vi "TrendsD06.vi"() -> ()   [LabVIEW 2019, in "D06.lvlib"]
uses:
  D06.lvlib
  <vilib>/measure/mamon.llb/Trigger Detection for 1 Channel.vi
  <vilib>/measure/NI_MAPro.lvlib
panel:
  out "No Change":bool
  out "Sudden Change":bool
  out "Decrease":bool
  out "Increase":bool
  out "Previous  ES":dbl
  out "Present  Speed":dbl
  out "Present Error":dbl format="%#.2g"
  out "Previous Error":dbl
  out "Previous  Speed":dbl
  out "Previous PW":dbl caption="Control Information"
  out "Pulse Trends":waveform(i16)[](graph) caption="Waveform Chart - Dark"
  in  "Close":bool
  out "disc name":string="Disc 06 Trends"
  out "dsgs":string="DSGS"
  out "Speed Trend":waveform(dbl)(graph) caption="Waveform Chart - Dark"
  out "Average Trend":waveform(dbl)[](graph) caption="Waveform Chart - Dark"
  out "Live Trend":waveform(dbl)[](graph) caption="Waveform Chart - Dark"
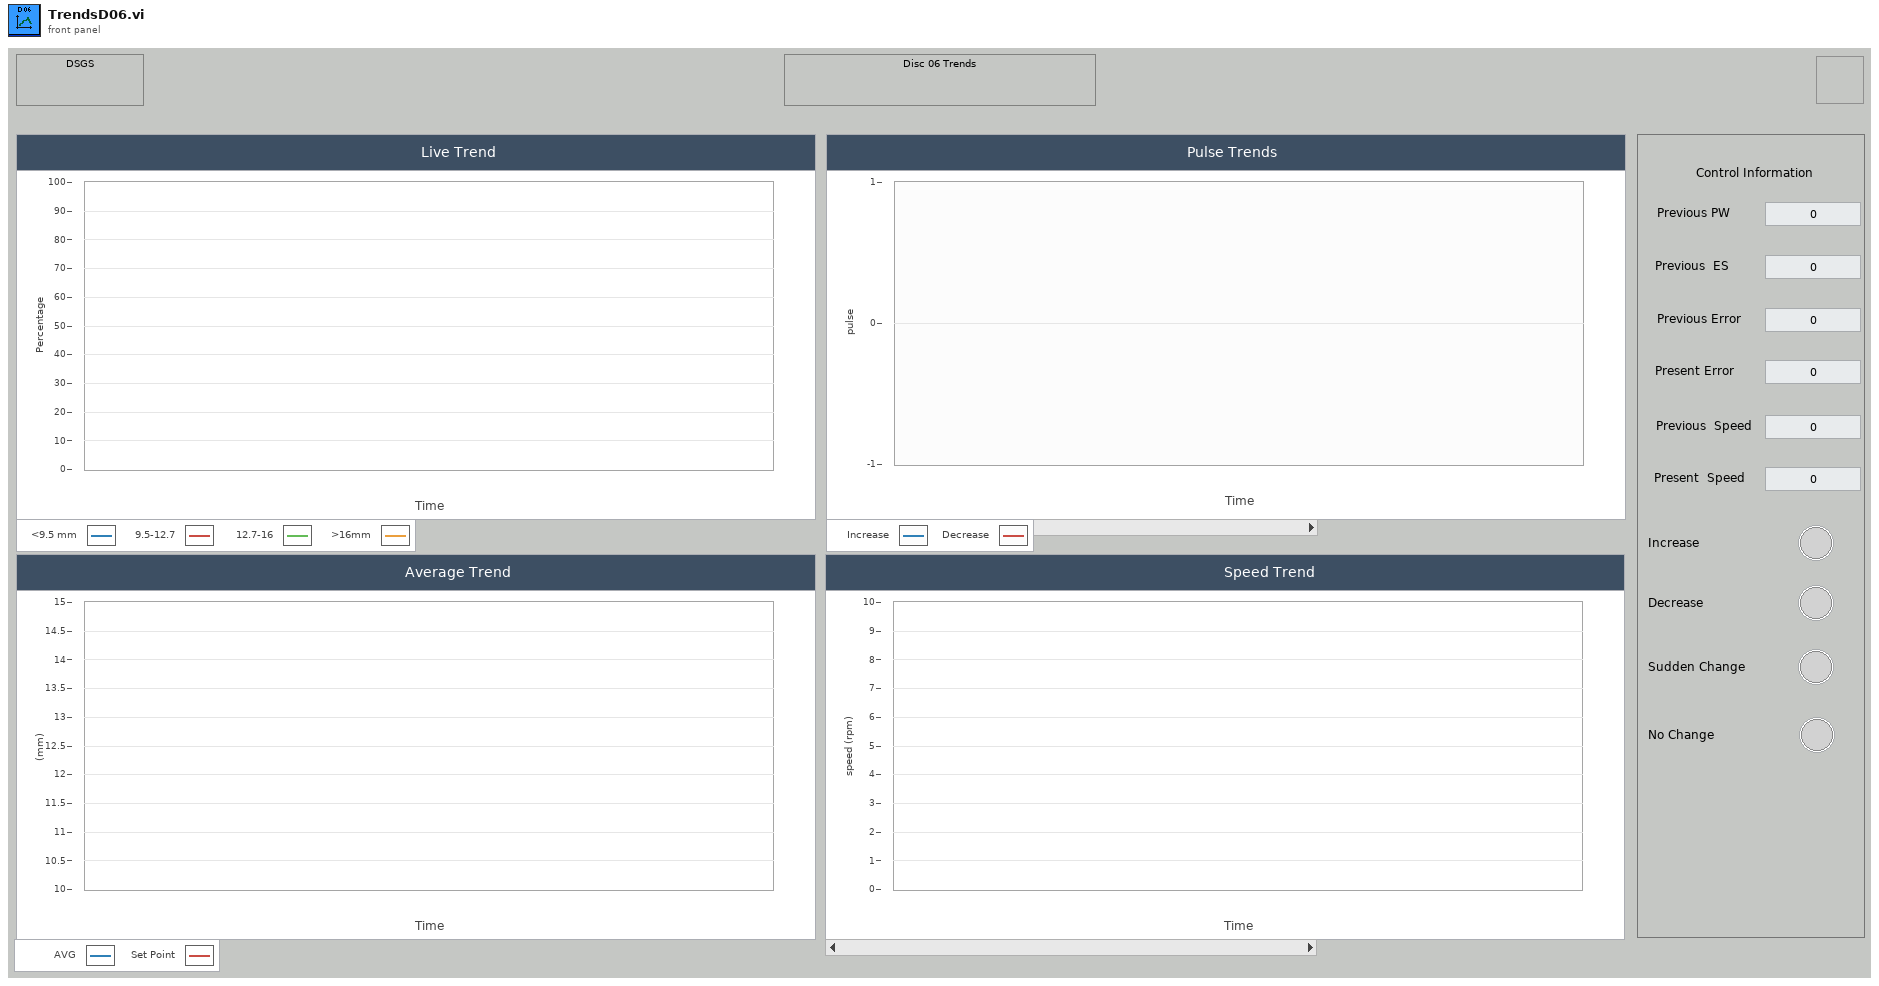
[diagram p1: front panel]
types:
  T1 = cluster{"decrease D06":bool, "increase D06":bool, "no change D06":bool, "sudden change D06":bool, "last error 06":dbl, "previouse speed D06":dbl, "pulse width D06":dbl, "slope D06":dbl}
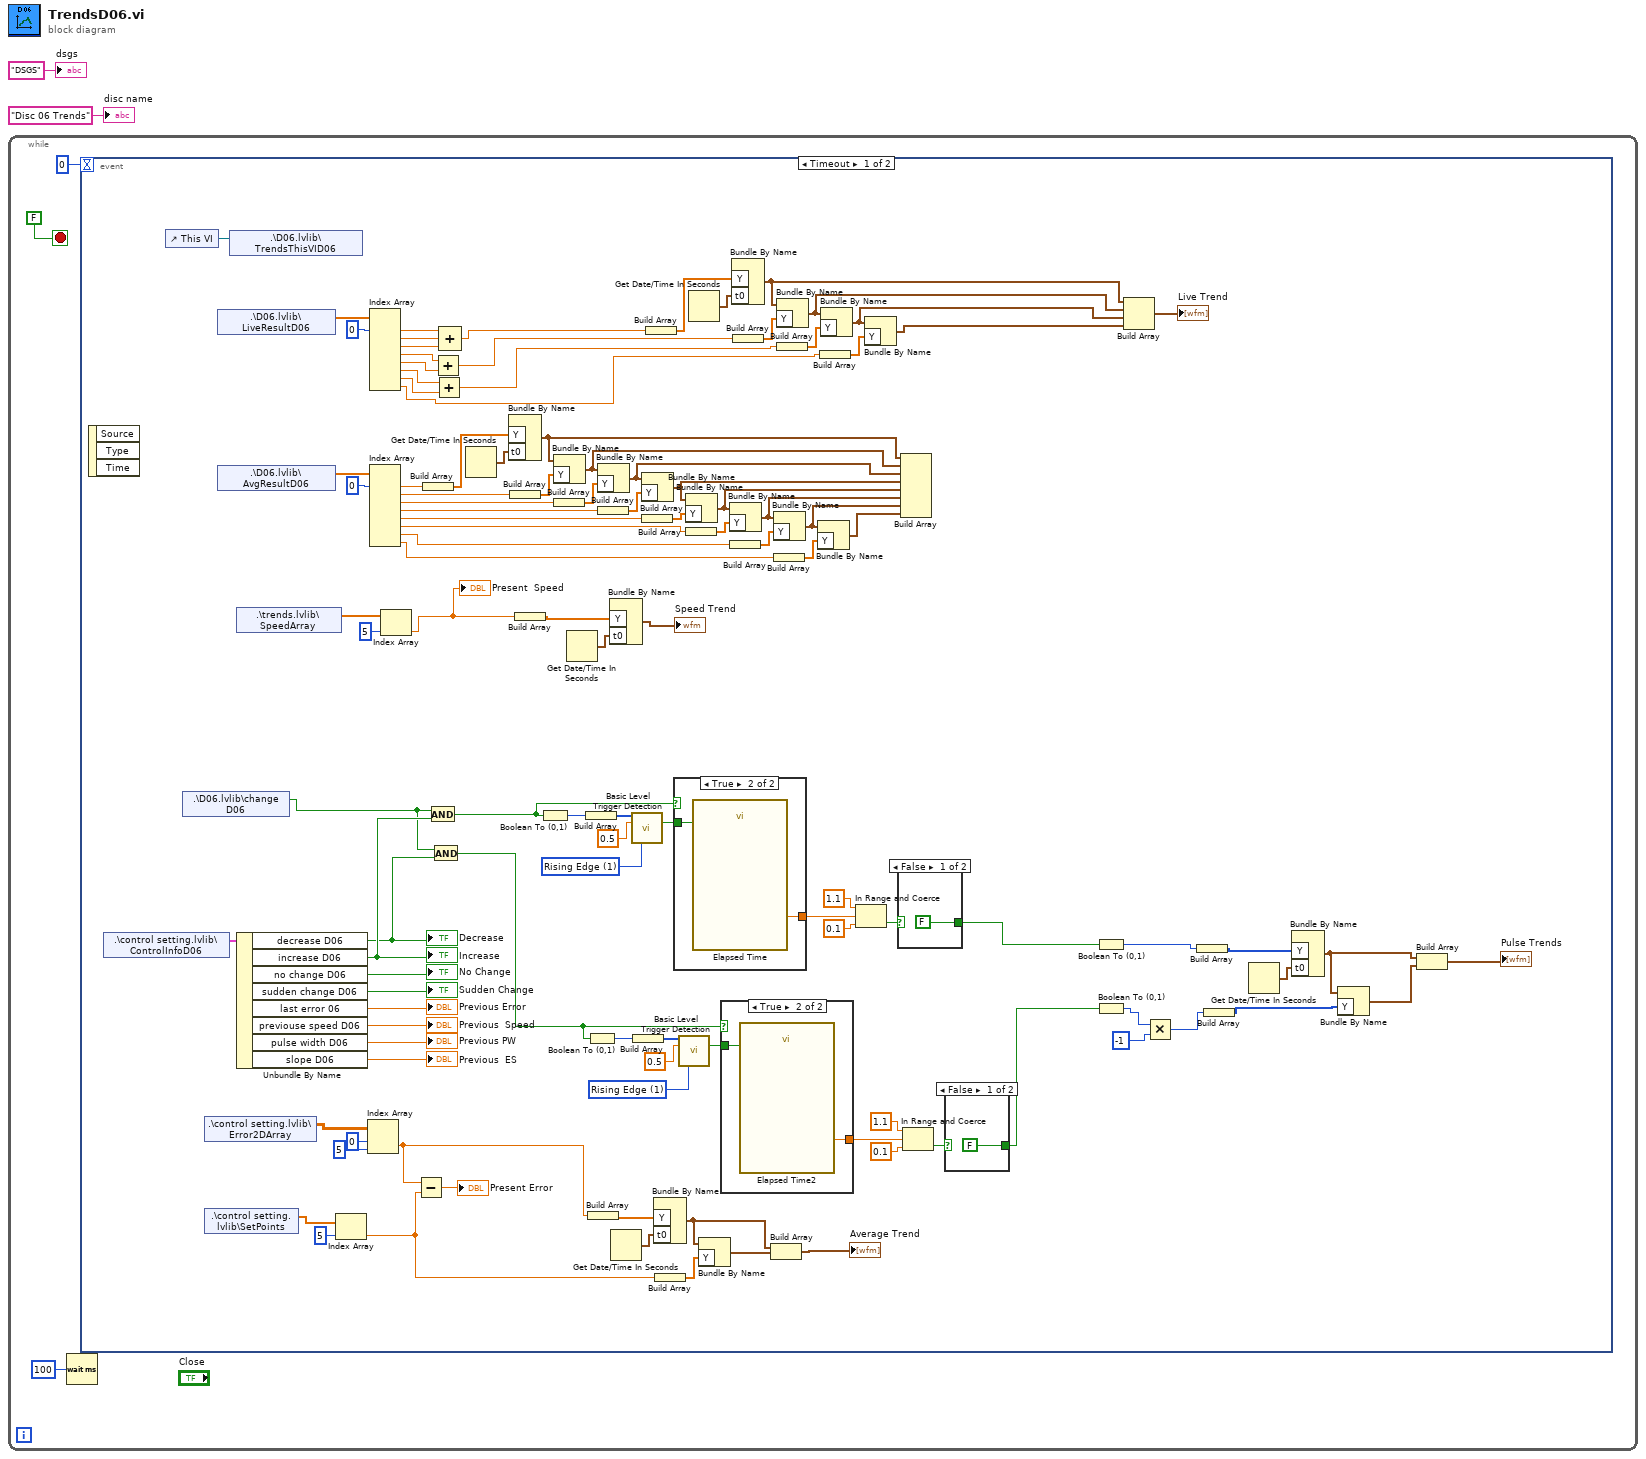
[diagram p0: block diagram]
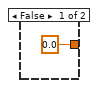
[diagram p2: hidden frame]
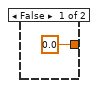
[diagram p4: hidden frame]
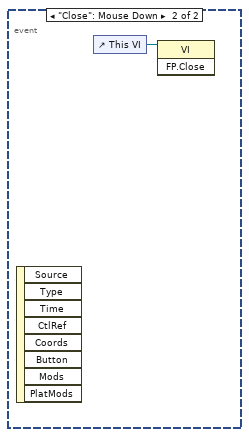
[diagram p6: hidden frame]
diagram:
  n1 = while {
    stop <- FALSE stop-if-true
    n2 = Wait (ms)(milliseconds to wait=u32 100) -> ()  [unwired: 1 out]
    n3 = event shown="[0] Timeout" {
      selector: _ -> [_ _]
      dyn-events: _ -> [_ _]
      timeout: 0 -> [_ _]
      event Timeout {
        w30 = u16 1 items=["Falling Edge", "Rising Edge"] ("trigger slope")
        w42 = u16 1 items=["Falling Edge", "Rising Edge"] ("trigger slope")
        n4 = event-data() -> ()  [unwired: 1 in, 3 out]
        n5 = shared-variable ".\\control setting.lvlib\\ControlInfoD06"() -> (w63:T1)  [unwired: 1 in, 1 out]
        n6 = control-ref of="This VI"() -> (w79:refnum<vi>)
        n7 = shared-variable ".\\D06.lvlib\\change D06"() -> (w28:bool)  [unwired: 1 in, 1 out]
        n8 = shared-variable ".\\control setting.lvlib\\Error2DArray"() -> (w56:dbl[][])  [unwired: 1 in, 1 out]
        n9 = shared-variable ".\\control setting.lvlib\\SetPoints"() -> (w53:dbl[])  [unwired: 1 in, 1 out]
        n10 = shared-variable ".\\D06.lvlib\\LiveResultD06"() -> (w118:dbl[])  [unwired: 1 in, 1 out]
        n11 = shared-variable ".\\D06.lvlib\\AvgResultD06"() -> (w85:dbl[])  [unwired: 1 in, 1 out]
        n12 = shared-variable ".\\D06.lvlib\\TrendsThisVID06"(w79) -> ()  [unwired: 1 in, 1 out]
        n13 = shared-variable ".\\trends.lvlib\\SpeedArray"() -> (w68:dbl[])  [unwired: 1 in, 1 out]
        n14 = Unbundle By Name(w63) -> ("decrease D06"=w27:bool, "increase D06"=w40:bool, "no change D06"=→"No Change":bool, "sudden change D06"=→"Sudden Change":bool, "last error 06"=→"Previous Error":dbl, "previouse speed D06"=→"Previous  Speed":dbl, "pulse width D06"=→"Previous PW":dbl, "slope D06"=→"Previous  ES":dbl)
        "Increase" <- w40
        "Decrease" <- w27
        n15 = Index Array(array=w53, index=5) -> (element=w9:dbl)
        n16 = Index Array(array=w56, index (row)=0, index (col)=5 ("disabled index (col)")) -> (element=w10:dbl)
        n17 = Index Array(array=w118, index #1=0 ("index")) -> (element #1=w24:dbl, element #2=w23:dbl, element #3=w22:dbl, element #4=w21:dbl, element #5=w20:dbl, element #6=w19:dbl, element #7=w18:dbl, element #8=w14:dbl)  [unwired: 7 in]
        n18 = Index Array(array=w85, index #1=0 ("index")) -> (element #1=w95:dbl, element #2=w96:dbl, element #3=w98:dbl, element #4=w100:dbl, element #5=w101:dbl, element #6=w103:dbl, element #7=w105:dbl, element #8=w82:dbl)  [unwired: 7 in]
        n19 = Index Array(array=w68, index=5) -> (element=w50:dbl)
        "Present  Speed" <- w50
        n20 = Subtract(x=w10, y=w9) -> (x-y=→"Present Error":dbl)
        n21 = Build Array(w95) -> (w106:dbl[])
        n22 = And(x=w28, y=w40) -> (x .and. y?=w39:bool)
        n23 = And(x=w28, y=w27) -> (x .and. y?=w26:bool)
        n24 = Add(x=w21, y=w20) -> (x+y=w16:dbl)
        n25 = Add(x=w19, y=w18) -> (x+y=w15:dbl)
        n26 = Compound Arithmetic op=ADD(w24, w23, w22) -> (w17:dbl)
        n27 = Get Date/Time In Seconds() -> (seconds since 1Jan1904=w88:timestamp)
        n28 = Bundle By Name("Y"=w106, "t0"=w88) -> (w94:waveform(dbl))  [unwired: 1 in]
        n29 = Build Array(w96) -> (w97:dbl[])
        n30 = Build Array(w50) -> (w66:dbl[])
        n31 = Boolean To (0,1)(Boolean=w39) -> (0, 1=w45:i16)
        n32 = Bundle By Name(cluster=w94, "Y"=w97) -> (w93:waveform(dbl))
        n33 = Build Array(w98) -> (w99:dbl[])
        n34 = Get Date/Time In Seconds() -> (seconds since 1Jan1904=w65:timestamp)
        n35 = Build Array(w45) -> (w44:i16[])
        n36 = Boolean To (0,1)(Boolean=w26) -> (0, 1=w33:i16)
        n37 = Build Array(w10) -> (w11:dbl[])
        n38 = Bundle By Name(cluster=w93, "Y"=w99) -> (w92:waveform(dbl))
        n39 = Build Array(w100) -> (w87:dbl[])
        n40 = Bundle By Name("Y"=w66, "t0"=w65) -> (→"Speed Trend":waveform(dbl))  [unwired: 1 in]
        n41 = Get Date/Time In Seconds() -> (seconds since 1Jan1904=w13:timestamp)
        n42 = call-poly <vilib>:"Basic Level Trigger Detection.vi"("signal in"=w44, "level"=0.5, "trigger slope"=w42) -> ("trigger detected?"=w41:bool)  [unwired: 10 in, 2 out]
        n43 = Build Array(w33) -> (w32:i16[])
        n44 = Bundle By Name(cluster=w92, "Y"=w87) -> (w91:waveform(dbl))
        n45 = Build Array(w101) -> (w102:dbl[])
        n46 = Build Array(w17) -> (w108:dbl[])
        n47 = Bundle By Name("Y"=w11, "t0"=w13) -> (w7:waveform(dbl))  [unwired: 1 in]
        n48 = Build Array(w9) -> (w12:dbl[])
        n49 = case shown="True" w39 {
          tunnel: [0.0 ("Elapsed Time (s)") w125] -> w49
          tunnel: w41 -> [_ w126]
          frame False {
          }
          frame True {
            n50 = call "Elapsed Time"("Reset"=w126) -> ("Elapsed Time (s)"=w125:dbl)  [unwired: 11 in, 7 out]
          }
        }
        n51 = call-poly <vilib>:"Basic Level Trigger Detection.vi"("signal in"=w32, "level"=0.5, "trigger slope"=w30) -> ("trigger detected?"=w29:bool)  [unwired: 10 in, 2 out]
        n52 = Bundle By Name(cluster=w91, "Y"=w102) -> (w90:waveform(dbl))
        n53 = Build Array(w103) -> (w104:dbl[])
        n54 = Get Date/Time In Seconds() -> (seconds since 1Jan1904=w115:timestamp)
        n55 = Bundle By Name(cluster=w7, "Y"=w12) -> (w8:waveform(dbl))
        n56 = case shown="True" w26 {
          tunnel: [0.0 ("Elapsed Time (s)") w120] -> w37
          tunnel: w29 -> [_ w121]
          frame False {
          }
          frame True {
            n57 = call "Elapsed Time2"("Reset"=w121) -> ("Elapsed Time (s)"=w120:dbl)  [unwired: 11 in, 7 out]
          }
        }
        n58 = Bundle By Name(cluster=w90, "Y"=w104) -> (w89:waveform(dbl))
        n59 = Build Array(w105) -> (w107:dbl[])
        n60 = Bundle By Name("Y"=w108, "t0"=w115) -> (w111:waveform(dbl))  [unwired: 1 in]
        n61 = Build Array(w16) -> (w110:dbl[])
        n62 = Build Array(w7, w8) -> (→"Average Trend":waveform(dbl)[])
        n63 = Bundle By Name(cluster=w89, "Y"=w107) -> (w83:waveform(dbl))
        n64 = Build Array(w82) -> (w84:dbl[])
        n65 = Bundle By Name(cluster=w111, "Y"=w110) -> (w112:waveform(dbl))
        n66 = Build Array(w15) -> (w109:dbl[])
        n67 = Bundle By Name(cluster=w83, "Y"=w84) -> (w81:waveform(dbl))
        n68 = Build Array(w14) -> (w116:dbl[])
        n69 = Bundle By Name(cluster=w112, "Y"=w109) -> (w113:waveform(dbl))
        n70 = In Range and Coerce(upper limit=1.1, x=w49, lower limit=0.1) -> (In Range?=w46:bool)  [unwired: 1 out]
        n71 = Bundle By Name(cluster=w113, "Y"=w116) -> (w114:waveform(dbl))
        n72 = case shown="False" w46 {
          selector: w46 -> [_ w128]
          tunnel: [FALSE w128] -> w38
          frame False {
          }
          frame True {
          }
        }
        n73 = Build Array(w94, w93, w92, w91, w90, w89, w83, w81) -> ()  [unwired: 1 out]
        n74 = In Range and Coerce(upper limit=1.1, x=w37, lower limit=0.1) -> (In Range?=w34:bool)  [unwired: 1 out]
        n75 = case shown="False" w34 {
          selector: w34 -> [_ w123]
          tunnel: [FALSE w123] -> w25
          frame False {
          }
          frame True {
          }
        }
        n76 = Boolean To (0,1)(Boolean=w38) -> (0, 1=w76:i16)
        n77 = Boolean To (0,1)(Boolean=w25) -> (0, 1=w72:i16)
        n78 = Build Array(w111, w112, w113, w114) -> (→"Live Trend":waveform(dbl)[])
        n79 = Multiply(x=w72, y=i16 -1 ("0, 1")) -> (x*y=w70:i16)
        n80 = Build Array(w76) -> (w77:i16[])
        n81 = Build Array(w70) -> (w75:i16[])
        n82 = Get Date/Time In Seconds() -> (seconds since 1Jan1904=w78:timestamp)
        n83 = Bundle By Name("Y"=w77, "t0"=w78) -> (w74:waveform(i16))  [unwired: 1 in]
        n84 = Bundle By Name(cluster=w74, "Y"=w75) -> (w73:waveform(i16))
        n85 = Build Array(w74, w73) -> (→"Pulse Trends":waveform(i16)[])
      }
      event "Close": Mouse Down {
        n86 = event-data() -> ()  [unwired: 1 in, 8 out]
        n87 = control-ref of="This VI"() -> (w129:refnum<vi>)
        n88 = invoke class="VI" method="FP.Close"(reference=w129) -> ()  [unwired: 2 in, 3 out]
      }
    }
  }
  "dsgs" <- "DSGS" ("dsgs")
  "disc name" <- "Disc 06 Trends" ("disc name")
